vi "update.vi"(8 "error in (no error)":errorcluster, 10 "model":refnum<class "Model.lvclass">, 11 "EnabledState in":refnum<class "EnabledState.lvclass">) -> (0 "error out":errorcluster, 2 "model 2":refnum<class "Model.lvclass">, 3 "EnabledState out":refnum<class "EnabledState.lvclass">)   [LabVIEW 2013, in "EnabledState.lvclass"]
uses:
  EnabledState.lvclass
  Model/Model/Model/Model.lvclass
  Typedefs/StateSelector.ctl
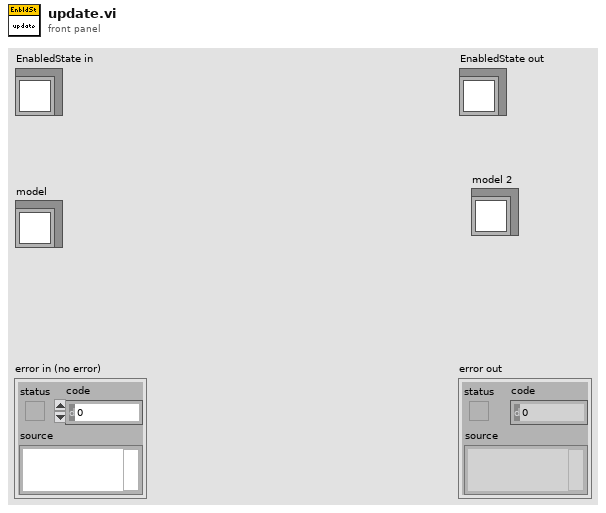
[diagram p1: front panel]
types:
  T1 = typedef "StateSelector.ctl" = enum16{"DataOnDemandState", "DataStreamingState", "FaultState", "OffState", "StandbyState"}
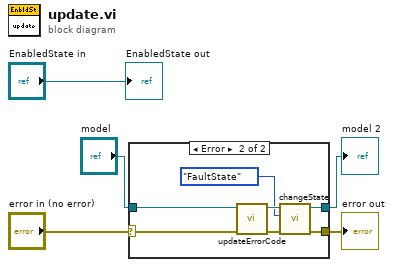
[diagram p0: block diagram]
diagram:
  n1 = case shown="Error" "error in (no error)" {
    selector: "error in (no error)" -> [w7 w14]
    tunnel: [w7 w10] -> w4
    tunnel: "model" -> [w6 w13]
    tunnel: [w6 w9] -> w1
    frame No Error {
    }
    frame Error {
      n2 = call "updateErrorCode.vi"("error in (no error)"=w14, "Model in"=w13) -> ("error out"=w11:errorcluster, "Model out"=w12:refnum<class "Model.lvclass">)  [unwired: 8 in]
      n3 = call "changeState.vi"("error in (no error)"=w11, "State:"=StateSelector."FaultState", "Model in"=w12) -> ("error out"=w10:errorcluster, "Model out"=w9:refnum<class "Model.lvclass">)  [unwired: 7 in]
    }
  }
  "error out" <- w4
  "model 2" <- w1
  "EnabledState out" <- "EnabledState in"
